vi "Move Log-Files.vi"(8 "error in":errorcluster, 10 "Force Move":bool, 11 "KIT-QVA in":refnum<class "KIT-QVA.lvclass">) -> (0 "error out":errorcluster, 3 "KIT-QVA out":refnum<class "KIT-QVA.lvclass">)   [LabVIEW 2016, in "KIT-QVA.lvlib" / "KIT-QVA.lvclass"]
doc: "When a quench occured, the logfiles on harddisk are moved to a timestamp-named folder."
uses:
  KIT-QVA.lvclass
  KIT-QVA.lvclass/KIT-QVA.ctl
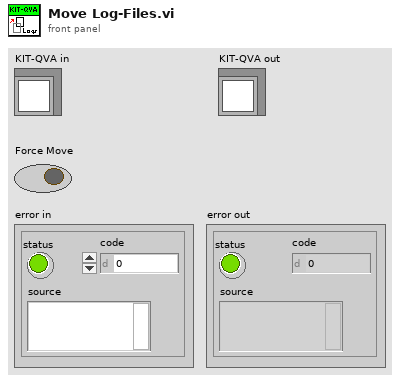
[diagram p1: front panel]
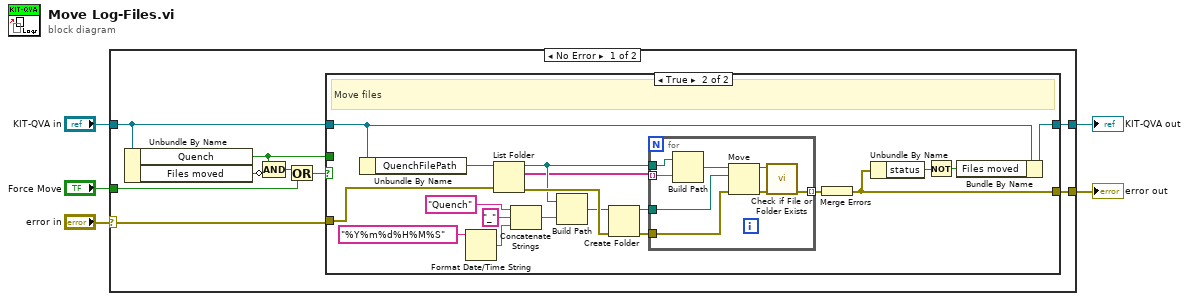
[diagram p0: block diagram]
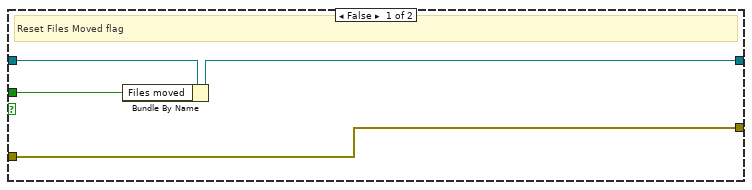
[diagram p2: hidden frame]
diagram:
  n1 = case shown="No Error" "error in" {
    selector: "error in" -> [w9 w47]
    tunnel: [w8 w47] -> w4
    tunnel: [w12 w46] -> w2
    tunnel: "KIT-QVA in" -> [w13 w46]
    tunnel: "Force Move" -> [w6 _]
    frame No Error {
      n2 = Unbundle By Name(w13) -> ("Quench"=w10:bool, "Files moved"=w14:bool)
      n3 = Compound Arithmetic op=AND(w10, invert w14) -> (w11:bool)
      n4 = Or(x=w11, y=w6) -> (x .or. y?=w7:bool)
      n5 = case shown="True" w7 {
        tunnel: w13 -> [w18 w24]
        tunnel: [w17 w37] -> w12
        tunnel: w10 -> [w16 _]
        tunnel: w9 -> [w15 w22]
        tunnel: [w15 w21] -> w8
        frame False {
          # "Reset Files Moved flag"
          n6 = Bundle By Name(cluster=w18, "Files moved"=w16) -> (w17:refnum<class "KIT-QVA.lvclass">)
        }
        frame True {
          # "Move files"
          n7 = Unbundle By Name(w24) -> ("QuenchFilePath"=w23:path)
          n8 = Format Date/Time String(time format string (%c)="%Y%m%d%H%M%S") -> (date/time string=w30:string)  [unwired: 2 in]
          n9 = List Folder(path=w23, error in=w22) -> (path out=w33:path, filenames=w32:string[], error out=w35:errorcluster)  [unwired: 2 in, 1 out]
          n10 = Concatenate Strings("Quench", "_" ("string"), w30) -> (w29:string)
          n11 = Build Path(base path=w33, name or relative path=w29) -> (appended path=w31:path)
          n12 = Create Folder(path (use dialog)=w31, error in=w35) -> (created path=w34:path, error out=w36:errorcluster)  [unwired: 1 in, 1 out]
          n13 = for {
            tunnel: w32 -> [w44] mode=indexing
            tunnel: w33 -> [w45]
            tunnel: w34 -> [w42]
            tunnel: w36 -> [w41]
            tunnel: [w38] -> w25 mode=indexing
            n14 = Build Path(base path=w45, name or relative path=w44) -> (appended path=w43:path)
            n15 = Move(source path=w43, error in=w41, 10:w42) -> (error out=w39:errorcluster, 3:w40:path)  [unwired: 2 in, 1 out]
            n16 = call <vilib>:"Check if File or Folder Exists.vi"("error in (no error)"=w39, "path"=w40) -> ("error out"=w38:errorcluster)  [unwired: 7 in, 2 out]
          }
          n17 = Merge Errors(w25) -> (w21:errorcluster)
          n18 = Unbundle By Name(w21) -> ("status"=w20:bool)
          n19 = Not(x=w20) -> (.not. x?=w19:bool)
          n20 = Bundle By Name(cluster=w24, "Files moved"=w19) -> (w37:refnum<class "KIT-QVA.lvclass">)
        }
      }
    }
    frame Error {
    }
  }
  "error out" <- w4
  "KIT-QVA out" <- w2
